vi "Create Module Config.vi"(8 "error in":errorcluster, 11 "DQMH Module Name":string) -> (0 "error out":errorcluster, 3 "config-ini out":refnum<class "config-ini.lvclass">)   [LabVIEW 2020, in "hse-config.lvlib" / "config-ini.lvclass"]
doc: "Loads the INI-file of an (HSE) DQMH module.\n\n____\nHAMPEL SOFTWARE ENGINEERING v3.8.0 (2023-12-18 14:41)"
uses:
  config-ini.lvclass
  hse-application/hse-application.lvclass
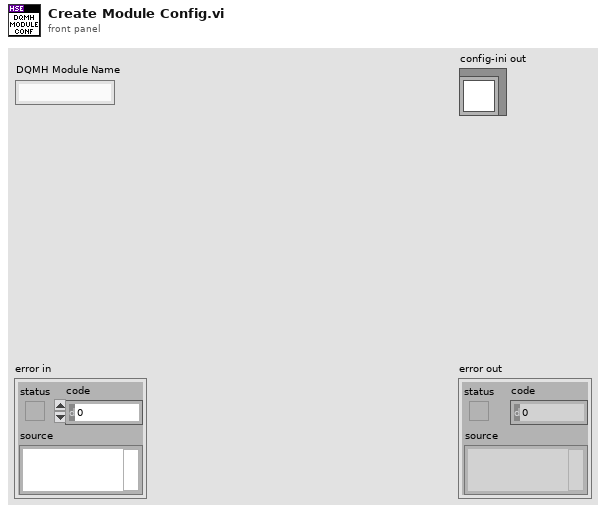
[diagram p1: front panel]
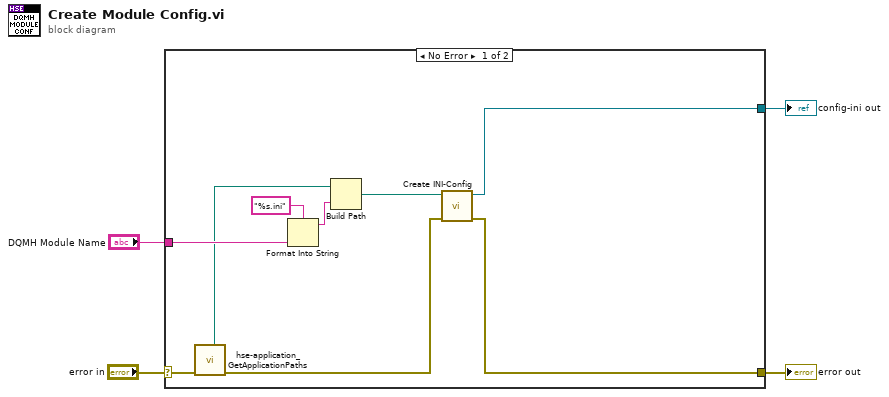
[diagram p0: block diagram]
diagram:
  n1 = case shown="No Error" "error in" {
    selector: "error in" -> [w13 w14]
    tunnel: [w6 w14] -> w3
    tunnel: [w5 _] -> w2
    tunnel: "DQMH Module Name" -> [w10 _]
    frame No Error {
      n2 = call "hse-application_GetApplicationPaths.vi"("error in"=w13) -> ("error out"=w7:errorcluster, "Config/Unit Directory"=w9:path)  [unwired: 4 in, 5 out]
      n3 = Format Into String(format string="%s.ini", w10) -> (resulting string=w12:string)  [unwired: 2 in, 1 out]
      n4 = Build Path(base path=w9, name or relative path=w12) -> (appended path=w8:path)
      n5 = call "Create INI-Config.vi"("error in"=w7, "INI Filepath"=w8) -> ("error out"=w6:errorcluster, "config-ini out"=w5:refnum<class "config-ini.lvclass">)  [unwired: 8 in]
    }
    frame Error {
    }
  }
  "error out" <- w3
  "config-ini out" <- w2
